vi "Main - Select Target and View.vi"   [LabVIEW 2013, in "GraphViz Mapping Visualizer.lvlib"]
uses:
  GraphViz Mapping Visualizer.lvlib
types:
  T1 = typedef "PLConfigurationSerializer.lvlib/engines cluster.ctl" = cluster{"engine configuration":refnum<class "engine configuration.lvclass">, "modules":refnum<class "TBM module configuration.lvclass">[]}
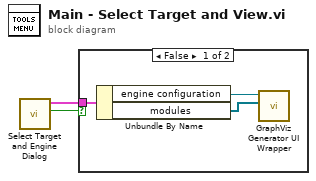
[diagram p0: block diagram]
diagram:
  n1 = call "Select Target and Engine Dialog.vi"() -> ("cancelled?"=w2:bool, "engines cluster"=w1:T1)  [unwired: 10 in]
  n2 = case shown="False" w2 {
    tunnel: w1 -> [w5 _]
    frame False {
      n3 = Unbundle By Name(w5) -> ("engine configuration"=w4:refnum<class "engine configuration.lvclass">, "modules"=w3:refnum<class "TBM module configuration.lvclass">[])
      n4 = call "GraphViz Generator UI Wrapper.vi"("Modules Configurations"=w3, "engine configuration in"=w4) -> ()  [unwired: 10 in]
    }
    frame True {
    }
  }
